vi "SLL DE DO Driver.vi"(6 "DO Channel Value Array":bool[](array[boolean]), 7 "DO Driver Option":T2=enum."Read Full Status", 8 "error in (no error)":errorcluster, 9 "DO Channel Value":bool, 10 "DO Channel Name Array":T1[](array[typedef]), 11 "DO Channel Name":T1) -> (0 "error out":errorcluster)   [LabVIEW 2013]
doc: "Copyright © 2005, Soliton Technologies.\nAll rights reserved."
uses:
  Controls/SLL DE DO Global Options.ctl
  Controls/SLL DE List of Digital Outputs.ctl
  Controls/SLL DE DAQ Global Options.ctl
  Controls/SLL DE DAQ Global Elements.ctl
  Controls/SLL DE DO Safe Value Global Options.ctl
  <vilib>/DAQmx/write.llb/DAQmx Write (Digital Bool 1Line 1Point).vi
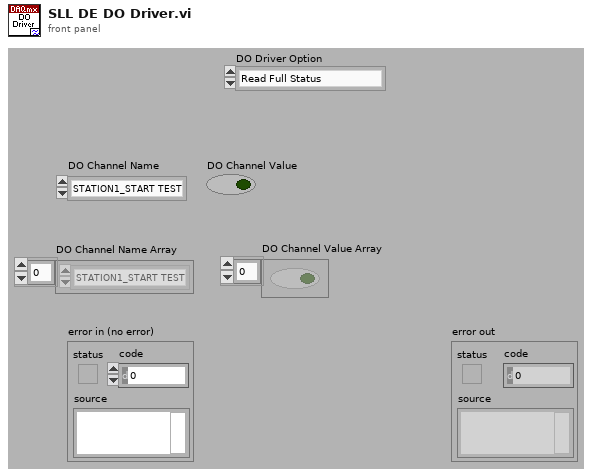
[diagram p1: front panel]
types:
  T1 = typedef "SLL DE List of Digital Outputs.ctl" = enum16{"STATION1_START TEST", "STATION1_STOP TEST", "STATION1_LIGHT1", "STATION1_LIGHT2", "STATION1_LIGHT3", "STATION1_SELECT_TEST", "STATION2_START TEST", "STATION2_STOP TEST", "STATION2_LIGHT1", "STATION2_LIGHT2", "STATION2_LIGHT3", "STATION2_SELECT_TEST", "STATION3_START TEST", "STATION3_STOP TEST", "STATION3_LIGHT1", "STATION3_LIGHT2", "STATION3_LIGHT3", "STATION3_SELECT_TEST", "STATION4_START TEST", "STATION4_STOP TEST", "STATION4_LIGHT1", "STATION4_LIGHT2", "STATION4_LIGHT3", "STATION4_SELECT_TEST"}
  T2 = typedef "SLL DE DO Global Options.ctl" = enum16{"Init", "Write Line", "Write Array", "Write Full Status", "Read Line", "Read Array", "Read Full Status", "Restart DO", "Send to Safe Mode", "Stop DO"}
  T3 = typedef "SLL DE DAQ Global Elements.ctl" = enum16{"AI Error", "AO Error", "DI Error", "DO Error", "AI Restart", "DI Restart", "AI Running", "AO Running", "DI Running", "DO Running", "DAQ Exit?"}
  T4 = typedef "SLL DE DAQ Global Options.ctl" = enum16{"Init", "Write 1", "Read 1", "Write Array", "Read Array", "Clear"}
  T5 = typedef "SLL DE DO Safe Value Global Options.ctl" = enum16{"Read", "Write"}
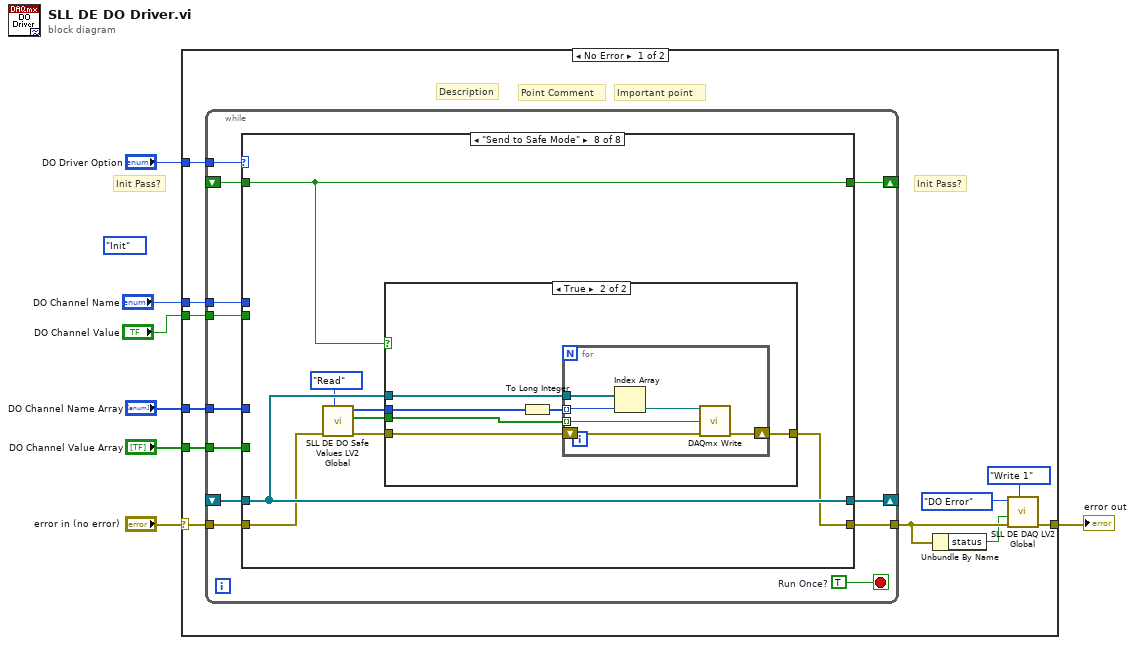
[diagram p0: block diagram]
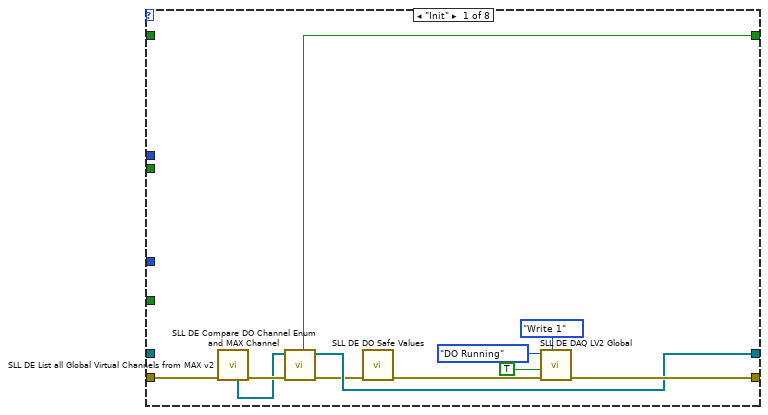
[diagram p2: hidden frame]
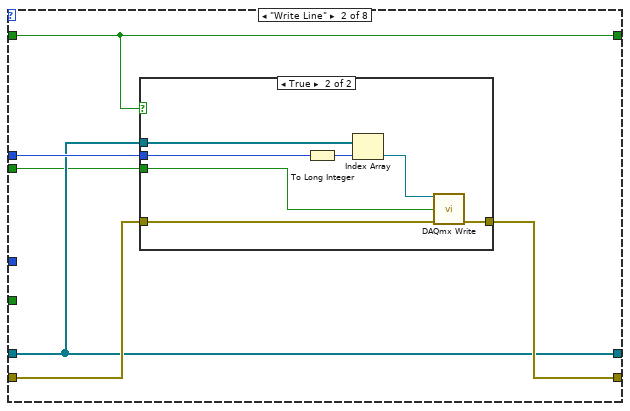
[diagram p3: hidden frame]
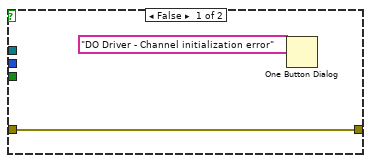
[diagram p4: hidden frame]
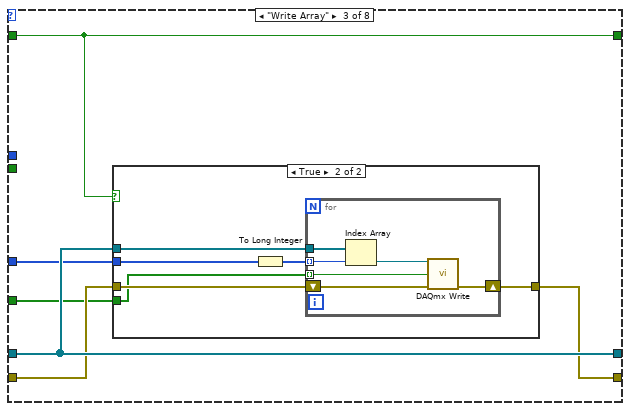
[diagram p5: hidden frame]
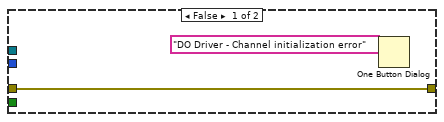
[diagram p6: hidden frame]
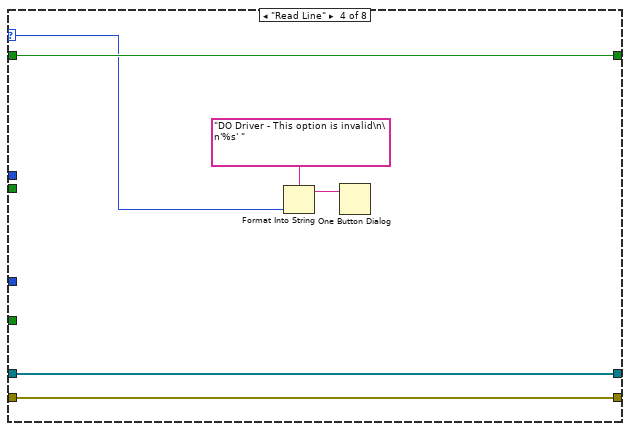
[diagram p7: hidden frame]
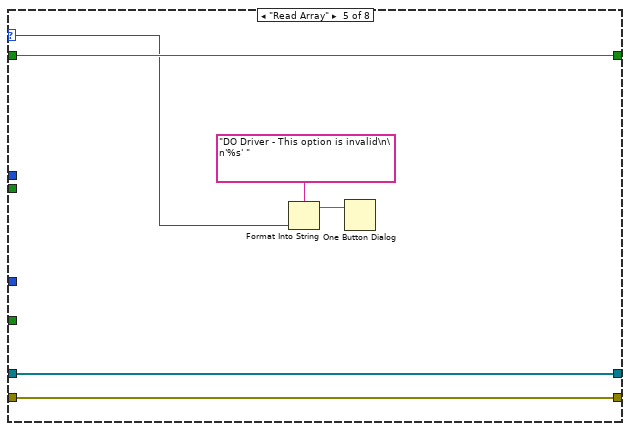
[diagram p8: hidden frame]
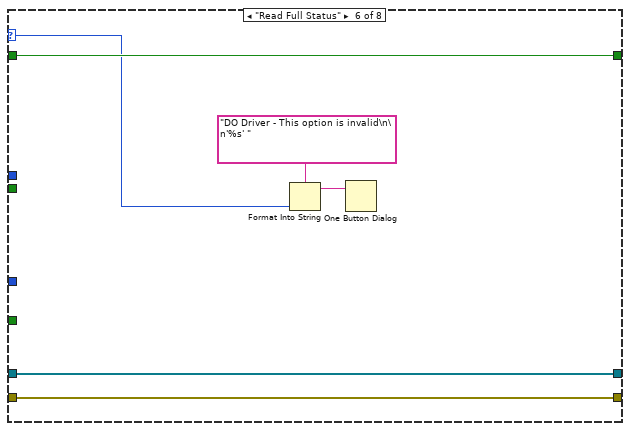
[diagram p9: hidden frame]
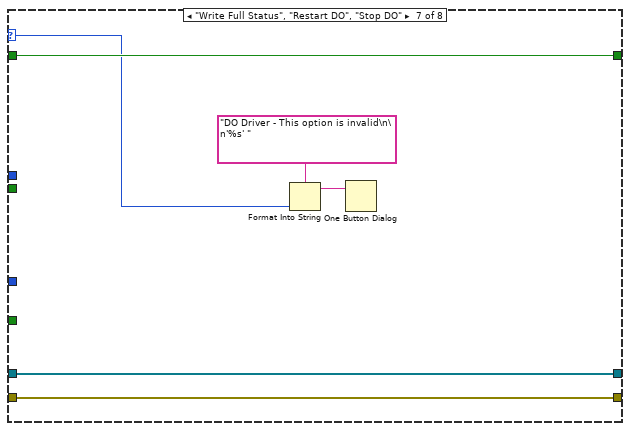
[diagram p10: hidden frame]
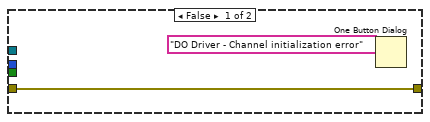
[diagram p11: hidden frame]
diagram:
  (unwired) SLL_DE_DO_Global_Options."Init" ("DO Driver Option 2")
  # "Init Pass?"
  n1 = case shown="No Error" "error in (no error)" {
    selector: "error in (no error)" -> [w18 w123]
    tunnel: [w10 w123] -> w6
    tunnel: "DO Driver Option" -> [w17 _]
    tunnel: "DO Channel Name" -> [w16 _]
    tunnel: "DO Channel Name Array" -> [w15 _]
    tunnel: "DO Channel Value" -> [w14 _]
    tunnel: "DO Channel Value Array" -> [w13 _]
    frame No Error {
      # "Init Pass?"
      # "Point Comment"
      # "Important point"
      # "Description"
      n2 = while {
        tunnel: w18 -> [w29]
        tunnel: [w28] -> w9
        shift-right: [w27] -> _
        shift-left: _ -> [w24]
        shift-right: [w26] -> _
        shift-left: _ -> [w23]
        tunnel: w17 -> [w25]
        tunnel: w16 -> [w22]
        tunnel: w15 -> [w21]
        tunnel: w14 -> [w20]
        tunnel: w13 -> [w19]
        stop <- w30 stop-if-true
        w30 = TRUE  # Run Once?
        n3 = case shown="\"Send to Safe Mode\"" w25 {
          selector: w25 -> [_ _ _ w77 w83 w89 w95 _]
          tunnel: w29 -> [w35 w47 w61 w80 w86 w92 w98 w104]
          tunnel: [w38 w46 w60 w80 w86 w92 w98 w106] -> w28
          tunnel: [w34 w42 w59 w81 w88 w94 w100 w107] -> w27
          tunnel: [w33 w44 w62 w82 w87 w93 w99 w108] -> w26
          tunnel: w24 -> [_ w42 w59 w81 w88 w94 w100 w107]
          tunnel: w23 -> [_ w44 w62 w82 w87 w93 w99 w108]
          tunnel: w22 -> [_ w45 _ _ _ _ _ _]
          tunnel: w21 -> [_ _ w58 _ _ _ _ _]
          tunnel: w20 -> [_ w43 _ _ _ _ _ _]
          tunnel: w19 -> [_ _ w57 _ _ _ _ _]
          frame "Init" {
            n4 = call "SLL DE List all Global Virtual Channels from MAX v2.vi"("error in (no error)"=w35) -> ("error out"=w37:errorcluster, "Digital Output"=w36:refnum<k21>[])  [unwired: 4 in, 5 out]
            n5 = call "SLL DE Compare DO Channel Enum and MAX Channel.vi"("error in (no error)"=w37, "Digital Output Channels"=w36) -> ("error out"=w32:errorcluster, "Channels Out"=w33:refnum<k21>[], "Pass?"=w34:bool)  [unwired: 7 in]
            n6 = call "SLL DE DO Safe Values.vi"("error in (no error)"=w32) -> ("error out"=w31:errorcluster)  [unwired: 8 in, 2 out]
            n7 = call "SLL DE DAQ LV2 Global.vi"("Option"=SLL_DE_DAQ_Global_Options."Write 1", "error in (no error)"=w31, "Status In"=TRUE, "Element"=SLL_DE_DAQ_Global_Elements."DO Running") -> ("error out"=w38:errorcluster)  [unwired: 5 in, 2 out]
          }
          frame "Write Line" {
            n8 = case shown="True" w42 {
              tunnel: w47 -> [w49 w53]
              tunnel: [w49 w52] -> w46
              tunnel: w45 -> [_ w54]
              tunnel: w44 -> [_ w56]
              tunnel: w43 -> [_ w50]
              frame False {
                n9 = One Button Dialog(message="DO Driver - Channel initialization error") -> ()  [unwired: 1 in, 1 out]
              }
              frame True {
                n10 = To Long Integer(number=w54) -> (32bit integer=w55:i32)
                n11 = Index Array(array=w56, index=w55) -> (element=w51:refnum<k21>)
                n12 = call-poly <vilib>:"DAQmx Write.vi"("task/channels in"=w51, "data"=w50, "error in"=w53) -> ("error out"=w52:errorcluster)  [unwired: 10 in, 2 out]
              }
            }
          }
          frame "Write Array" {
            n13 = case shown="True" w59 {
              tunnel: w61 -> [w64 w66]
              tunnel: [w64 w70] -> w60
              tunnel: w58 -> [_ w67]
              tunnel: w62 -> [_ w69]
              tunnel: w57 -> [_ w65]
              frame False {
                n14 = One Button Dialog(message="DO Driver - Channel initialization error") -> ()  [unwired: 1 in, 1 out]
              }
              frame True {
                n15 = To Long Integer(number=w67) -> (32bit integer=w68:i32[])
                n16 = for {
                  tunnel: w68 -> [w76] mode=indexing
                  tunnel: w69 -> [w75]
                  tunnel: w65 -> [w71] mode=indexing
                  shift-right: [w72] -> w70
                  shift-left: w66 -> [w73]
                  n17 = Index Array(array=w75, index=w76) -> (element=w74:refnum<k21>)
                  n18 = call-poly <vilib>:"DAQmx Write.vi"("task/channels in"=w74, "data"=w71, "error in"=w73) -> ("error out"=w72:errorcluster)  [unwired: 10 in, 2 out]
                }
              }
            }
          }
          frame "Read Line" {
            n19 = Format Into String(format string="DO Driver - This option is invalid\n\n'%s' " ("message"), w77) -> (resulting string=w78:string)  [unwired: 2 in, 1 out]
            n20 = One Button Dialog(message=w78) -> ()  [unwired: 1 in, 1 out]
          }
          frame "Read Array" {
            n21 = Format Into String(format string="DO Driver - This option is invalid\n\n'%s' " ("message"), w83) -> (resulting string=w84:string)  [unwired: 2 in, 1 out]
            n22 = One Button Dialog(message=w84) -> ()  [unwired: 1 in, 1 out]
          }
          frame "Read Full Status" {
            n23 = Format Into String(format string="DO Driver - This option is invalid\n\n'%s' " ("message"), w89) -> (resulting string=w90:string)  [unwired: 2 in, 1 out]
            n24 = One Button Dialog(message=w90) -> ()  [unwired: 1 in, 1 out]
          }
          frame "Write Full Status", "Restart DO", "Stop DO" {
            n25 = Format Into String(format string="DO Driver - This option is invalid\n\n'%s' " ("message"), w95) -> (resulting string=w96:string)  [unwired: 2 in, 1 out]
            n26 = One Button Dialog(message=w96) -> ()  [unwired: 1 in, 1 out]
          }
          frame "Send to Safe Mode" {
            n27 = call "SLL DE DO Safe Values LV2 Global.vi"("Cases"=SLL_DE_DO_Safe_Value_Global_Options."Read", "error in (no error)"=w104) -> ("error out"=w103:errorcluster, "Value Array Out"=w102:bool[], "Elements Out"=w101:T1[])  [unwired: 7 in]
            n28 = case shown="True" w107 {
              tunnel: w103 -> [w110 w112]
              tunnel: [w110 w116] -> w106
              tunnel: w101 -> [_ w113]
              tunnel: w108 -> [_ w115]
              tunnel: w102 -> [_ w111]
              frame False {
                n29 = One Button Dialog(message="DO Driver - Channel initialization error") -> ()  [unwired: 1 in, 1 out]
              }
              frame True {
                n30 = To Long Integer(number=w113) -> (32bit integer=w114:i32[])
                n31 = for {
                  tunnel: w114 -> [w122] mode=indexing
                  tunnel: w115 -> [w121]
                  tunnel: w111 -> [w117] mode=indexing
                  shift-right: [w118] -> w116
                  shift-left: w112 -> [w119]
                  n32 = Index Array(array=w121, index=w122) -> (element=w120:refnum<k21>)
                  n33 = call-poly <vilib>:"DAQmx Write.vi"("task/channels in"=w120, "data"=w117, "error in"=w119) -> ("error out"=w118:errorcluster)  [unwired: 10 in, 2 out]
                }
              }
            }
          }
        }
      }
      n34 = Unbundle By Name(w9) -> ("status"=w8:bool)
      n35 = call "SLL DE DAQ LV2 Global.vi"("Option"=SLL_DE_DAQ_Global_Options."Write 1", "error in (no error)"=w9, "Status In"=w8, "Element"=SLL_DE_DAQ_Global_Elements."DO Error") -> ("error out"=w10:errorcluster)  [unwired: 5 in, 2 out]
    }
    frame Error {
    }
  }
  "error out" <- w6
